vi "配置初始化.vi"(8 "error in (no error)":errorcluster) -> (0 "error out":errorcluster)   [LabVIEW 2016]
uses:
  <vilib>/Utility/config.llb/NI_LVConfig.lvlib
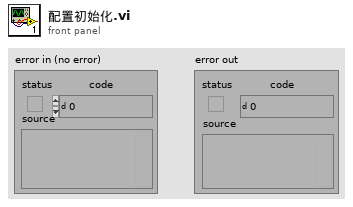
[diagram p1: front panel]
types:
  T1 = typedef "NI_LVConfig.lvlib/Config Data RefNum.ctl" = refnum<k1>
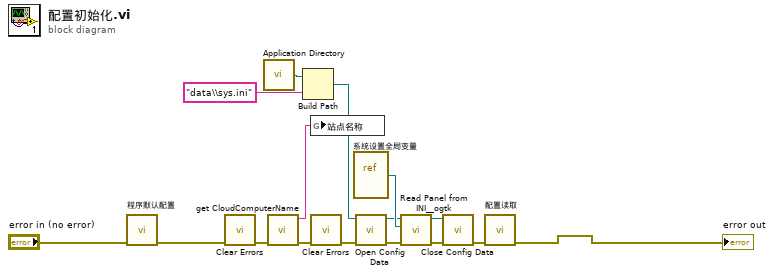
[diagram p0: block diagram]
diagram:
  n1 = call "程序默认配置.vi"("error in (no error)"="error in (no error)") -> ("error out"=w5:errorcluster)  [unwired: 10 in]
  n2 = call <vilib>:"Clear Errors.vi"("error in (no error)"=w5) -> ("error out"=w4:errorcluster)  [unwired: 5 in, 1 out]
  n3 = call <vilib>:"Application Directory.vi"() -> ("Application Directory"=w14:path)
  n4 = call "get CloudComputerName.vi"("error in (no error)"=w4) -> ("error out"=w6:errorcluster, "String/Binary data"=w7:string)  [unwired: 9 in]
  n5 = Build Path(base path=w14, name or relative path="data\\sys.ini" ("名称或相对路径")) -> (appended path=w16:path)
  n6 = global write "非断电保持全局变量.vi" "站点名称"(w7) -> ()
  n7 = call <vilib>:"Clear Errors.vi"("error in (no error)"=w6) -> ("error out"=w2:errorcluster)  [unwired: 5 in, 1 out]
  n8 = vi-ref "系统设置全局变量.vi"() -> (w11:refnum<vi>)
  n9 = call <vilib>:"Open Config Data.vi"("error in (no error)"=w2, "configuration file path"=w16) -> ("error out"=w9:errorcluster, "refnum"=w10:T1)  [unwired: 7 in, 1 out]
  n10 = call <userlib>:"Read Panel from INI__ogtk.vi"("error in (no error)"=w9, "VI ref"=w11, "refnum"=w10) -> ("error out"=w12:errorcluster, "refnum out"=w13:T1)  [unwired: 7 in]
  n11 = call <vilib>:"Close Config Data.vi"("error in (no error)"=w12, "refnum"=w13) -> ("error out"=w3:errorcluster)  [unwired: 8 in, 1 out]
  n12 = call "配置读取.vi"("error in (no error)"=w3) -> ("error out"=→"error out":errorcluster)  [unwired: 10 in]
